vi "PanelWizard_ResolveRelativePath.vi"(1 "Relative Path":path) -> (0 "Absolute  Path":path)   [LabVIEW 2012, in "PanelWizard.xctl"]
uses:
  PanelWizard.xctl
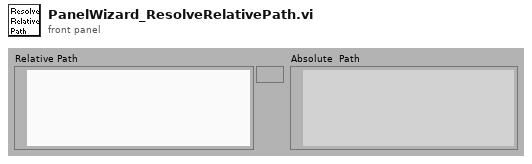
[diagram p1: front panel]
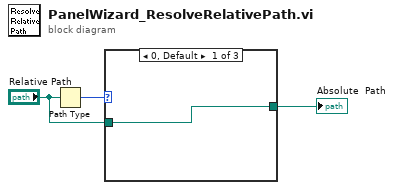
[diagram p0: block diagram]
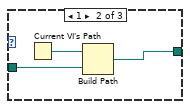
[diagram p2: hidden frame]
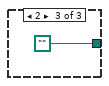
[diagram p3: hidden frame]
diagram:
  n1 = Path Type(1:"Relative Path") -> (0:w3:i16)
  n2 = case shown="0, Default" w3 {
    tunnel: [w4 w6 path ""] -> w2
    tunnel: "Relative Path" -> [w4 w7 _]
    frame 0, Default {
    }
    frame 1 {
      n3 = Current VI's Path() -> (path=w5:path)
      n4 = Build Path(base path=w5, name or relative path=w7) -> (appended path=w6:path)
    }
    frame 2 {
    }
  }
  "Absolute  Path" <- w2
